vi "BotSpeak_Wait.vi"(2 "Wait (sec)":dbl=1.0, 3 "Bot Settings":T1) -> (1 "Bot Settings":T1)   [LabVIEW 2012]
doc: "Causes VI to wait the specified number of seconds."
uses:
  <userlib>/botspeak/VIs/Direct/BotSpeak_Control.ctl
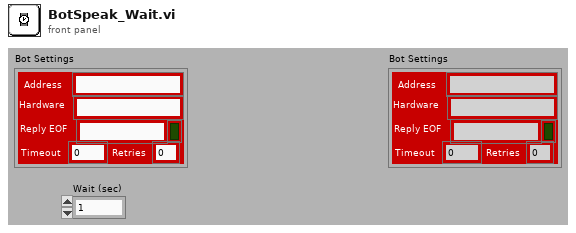
[diagram p1: front panel]
types:
  T1 = typedef "BotSpeak_Control.ctl" = cluster{"Address":string, "Reply EOF":string, "Hardware":string, "Retries":i8, "Timeout":i32, "Open?":bool}
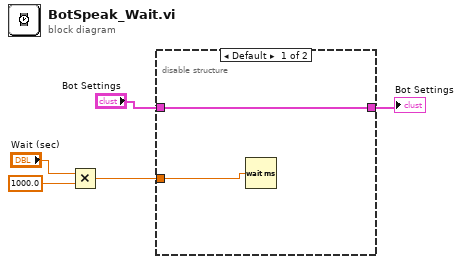
[diagram p0: block diagram]
diagram:
  n1 = Multiply(x="Wait (sec)", y=1000.0) -> (x*y=w3:dbl)
  n2 = disable-structure shown="Default" {
    disable-tunnel: w3 -> [w7 _]
    disable-tunnel: [w6 _] -> w1
    disable-tunnel: "Bot Settings" -> [w6 _]
    frame condition #0 (active) {
      n3 = Wait (ms)(milliseconds to wait=w7) -> ()  [unwired: 1 out]
    }
    frame condition #1 {
    }
  }
  "Bot Settings" <- w1
